vi "Graph_2ch.vi"(0 "Buff Len":i32=2, 1 "ch2":dbl format="%#.2g", 2 "ch1":dbl format="%#.2g", 3 "num in":i32=2, 6 "ArrayIn":T1(array[cluster])) -> (4 "num out":i32, 5 "Arr Out":T1(graph))   [LabVIEW 2017]
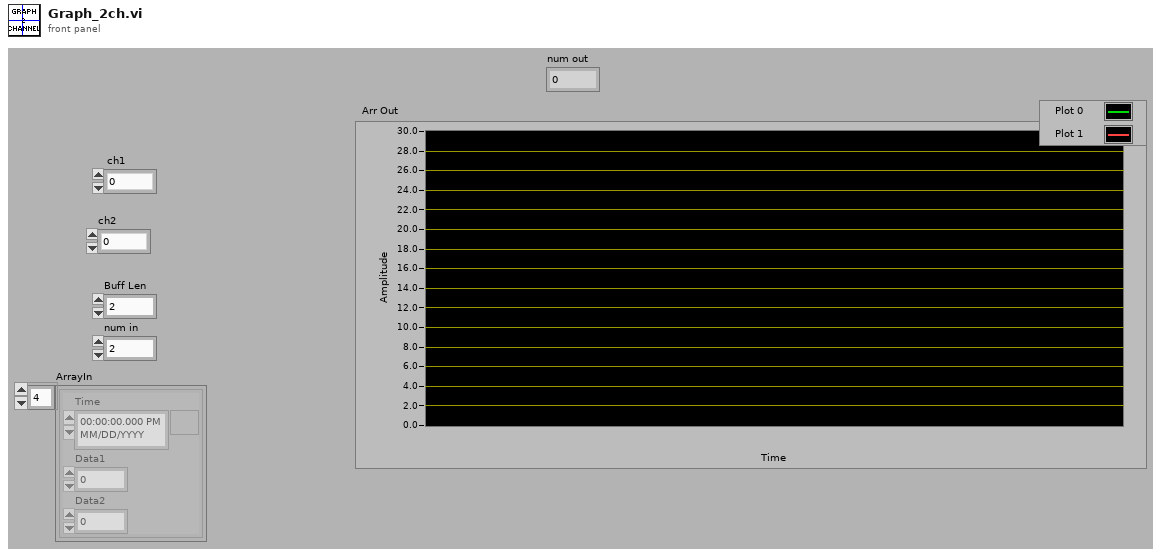
[diagram p1: front panel]
types:
  T1 = cluster{"Time":timestamp, "Data1":dbl, "Data2":dbl}[]
  T2 = cluster{"Time":timestamp, "Data1":dbl, "Data2":dbl}
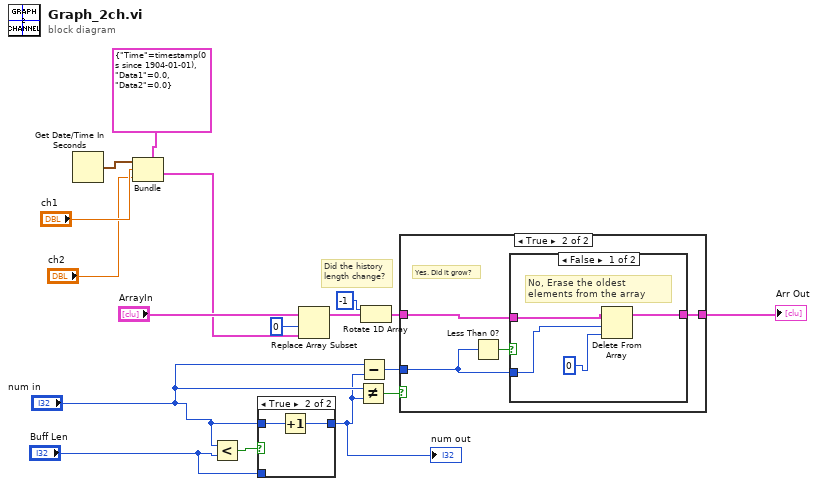
[diagram p0: block diagram]
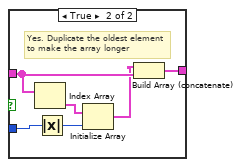
[diagram p4: hidden frame]
diagram:
  # "Did the history length change?"
  n1 = Get Date/Time In Seconds() -> (seconds since 1Jan1904=w17:timestamp)
  n2 = Bundle(cluster=T2 {"Time"=timestamp(0 s since 1904-01-01), "Data1"=0.0, "Data2"=0.0}, "Time"=w17, "Data1"="ch1", "Data2"="ch2") -> (w1:T2)
  n3 = Less?(x="num in", y="Buff Len") -> (x < y?=w10:bool)
  n4 = case shown="True" w10 {
    tunnel: "Buff Len" -> [w18 _]
    tunnel: [w18 w20] -> w4
    tunnel: "num in" -> [_ w19]
    frame False {
    }
    frame True {
      n5 = Increment(x=w19) -> (x+1=w20:i32)
    }
  }
  "num out" <- w4
  n6 = Replace Array Subset(array="ArrayIn", new element=w1, index=0) -> (w8:T1)
  n7 = Not Equal?(x="num in", y=w4) -> (x != y?=w14:bool)
  n8 = Subtract(x="num in", y=w4) -> (x-y=w5:i32)
  n9 = Rotate 1D Array(1:w8, 2:-1 ("n")) -> (0:w11:T1)
  n10 = case shown="True" w14 {
    tunnel: w11 -> [w21 w23]
    tunnel: [w21 w22] -> w6
    tunnel: w5 -> [_ w24]
    frame False {
      # "No. Do nothing"
    }
    frame True {
      # "Yes. Did it grow?"
      n11 = Less Than 0?(x=w24) -> (x < 0?=w25:bool)
      n12 = case shown="False" w25 {
        tunnel: w24 -> [w26 w33]
        tunnel: w23 -> [w29 w31]
        tunnel: [w28 w34] -> w22
        frame False {
          # "No, Erase the oldest elements from the array"
          n13 = Delete From Array(array=w29, length=w26, index=0) -> (array with subset deleted=w28:T1)  [unwired: 1 out]
        }
        frame True {
          # "Yes. Duplicate the oldest element to make the array longer"
          n14 = Index Array(array=w31) -> (element=w35:T2)  [unwired: 1 in]
          n15 = Absolute Value(x=w33) -> (abs(x)=w32:i32)
          n16 = Initialize Array(w35, w32) -> (w30:T1)
          n17 = Build Array (concatenate)(w30, w31) -> (w34:T1)
        }
      }
    }
  }
  "Arr Out" <- w6
